vi "FitCurveCorrelation.vi"() -> ()   [LabVIEW 2010]
uses:
  <vilib>/Analysis/1siggen.llb/Ramp Pattern by Samples.vi
  <vilib>/gmath/NumericalOptimization/Nonlinear Curve Fit LM.vi
  <vilib>/gmath/NI_Gmath.lvlib
  <vilib>/Analysis/NI_AALBase.lvlib
panel:
  out "error out":errorcluster
  out "Correlation Matrix":string[][](table)
  out "BestFit":cluster{"Name":string, "Parameter":dbl}[](array[cluster]) caption="Parameter Name          best Fit" {"Parameter" format="%.6f"}
  in  "Guess":T1(array[cluster])=[{"Name"="Offset", "Value"=0.0, "Fit?"=TRUE}, {"Name"="Ampl. 1", "Value"=2.0, "Fit?"=TRUE}, {"Name"="TC 1", "Value"=0.1, "Fit?"=TRUE}, {"Name"="Ampl. 2", "Value"=2.0, "Fit?"=TRUE}, {"Name"="TC 2", "Value"=0.3, "Fit?"=TRUE}] caption="Parameter Name     Guess        Fit?"
  in  "Noise":dbl=0.02
  in  "Simulation parameters":dbl[](array[numeric])=[0.2, 2.0, 0.02, 1.5, 0.2] caption="Offset\n\nAmplitude 1\n\nTime constant 1\n\nAmplitude 2\n\nTime  constant 2"
  in  "stop":bool
  out "XY Graph":cluster{cdb[]}[](graph)
  # "This demo simulates noisy data\nReplace with your experimental data!"
  # "- Run VI\n- Change simulation parameters\n- Change Noise\n- Change Guess\n- enable or disable fitting for some\n   parameters\n\n- Watch the quality of the fit."
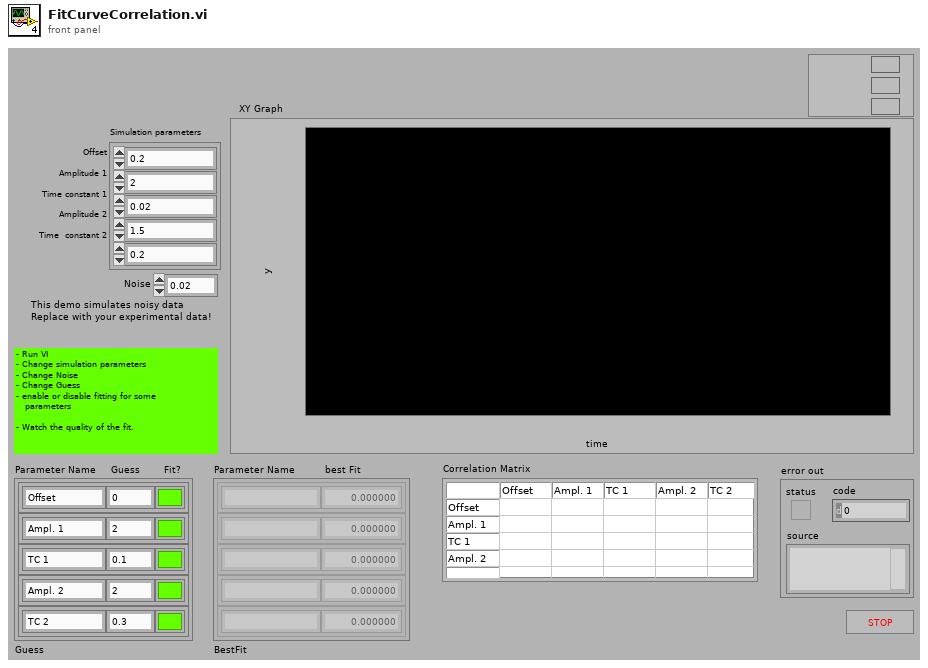
[diagram p1: front panel]
types:
  T1 = cluster{"Name":string, "Value":dbl, "Fit?":bool}[]
  T2 = typedef "NI_Matrix.lvlib/RealMatrix.ctl" = dbl[][]
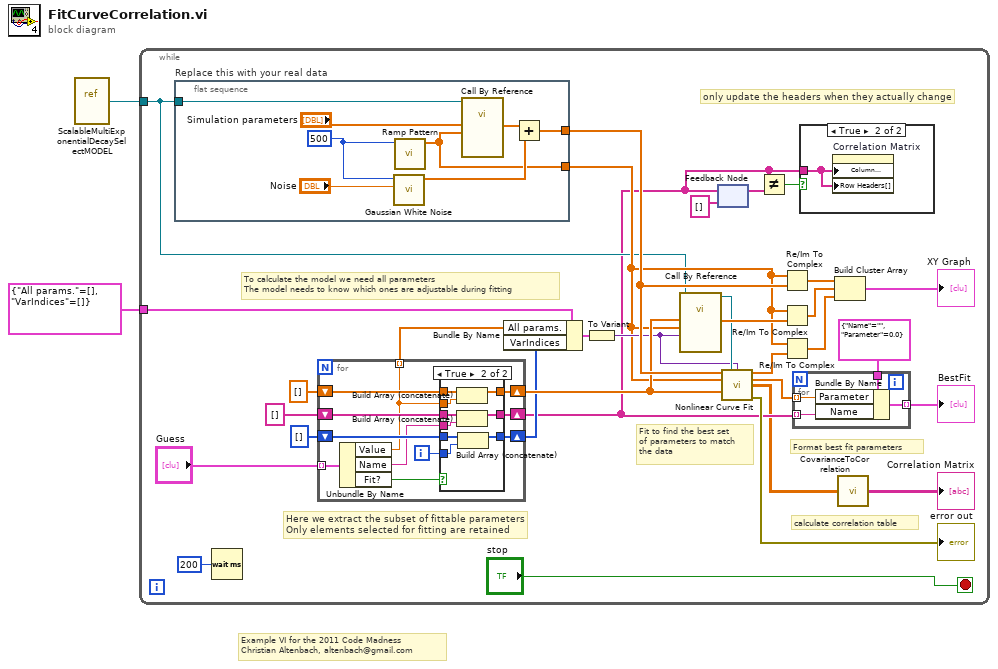
[diagram p0: block diagram]
diagram:
  # "Example VI for the 2011 Code Madness\nChristian Altenbach, altenbach@gmail.com"
  n1 = vi-ref "ScalableMultiExponentialDecaySelectMODEL.vi"() -> (w2:refnum<vi>)
  n2 = while {
    tunnel: w2 -> [w11]
    tunnel: cluster{"All params.":dbl[], "VarIndices":i32[]} {"All params."=[], "VarIndices"=[]} -> [w10]
    stop <- "stop" stop-if-true
    # "calculate correlation table"
    # "only update the headers when they actually change"
    # "Fit to find the best set\nof parameters to match\nthe data"
    # "Format best fit parameters"
    # "To calculate the model we need all parameters\nThe model needs to know which ones are adjustable during fitting"
    # "Here we extract the subset of fittable parameters\nOnly elements selected for fitting are retained"
    n3 = flat-sequence "Replace this with your real data" {
      tunnel: [w39] -> w25
      tunnel: [w37] -> w12
      tunnel: w11 -> [w36]
      frame #0 {
        w43 = 500 ("samples")
        n4 = call <vilib>:"Gaussian White Noise.vi"("standard deviation"="Noise", "samples"=w43) -> ("Gaussian noise pattern"=w41:dbl[])  [unwired: 8 in, 1 out]
        n5 = call-poly <vilib>:"Ramp Pattern.vi"("samples"=w43) -> ("Ramp Pattern"=w37:dbl[])  [unwired: 9 in, 1 out]
        n6 = call-by-ref "?"(reference=w36, "frequency"=w37, "tau"="Simulation parameters") -> ("Phase"=w42:dbl[])  [unwired: 3 in, 4 out]
        n7 = Add(x=w42, y=w41) -> (x+y=w39:dbl[])
      }
    }
    n8 = Wait (ms)(milliseconds to wait=u32 200) -> ()  [unwired: 1 out]
    n9 = for {
      shift-right: [w58] -> w23
      shift-left: dbl[] [] -> [w57]
      tunnel: "Guess" -> [w56] mode=indexing
      tunnel: [w49] -> w20 mode=indexing
      shift-right: [w54] -> w19
      shift-left: i32[] [] -> [w53]
      shift-right: [w50] -> w5
      shift-left: string[] [] -> [w51]
      i -> [w52]
      n10 = Unbundle By Name(w56) -> ("Value"=w49:dbl, "Name"=w48:string, "Fit?"=w55:bool)
      n11 = case shown="True" w55 {
        tunnel: [w61 w69] -> w58
        tunnel: w57 -> [w61 w70]
        tunnel: w49 -> [_ w68]
        tunnel: [w60 w67] -> w54
        tunnel: w53 -> [w60 w66]
        tunnel: w52 -> [_ w65]
        tunnel: [w59 w63] -> w50
        tunnel: w51 -> [w59 w64]
        tunnel: w48 -> [_ w62]
        frame False {
        }
        frame True {
          n12 = Build Array (concatenate)(w70, w68) -> (w69:dbl[])
          n13 = Build Array (concatenate)(w64, w62) -> (w63:string[])
          n14 = Build Array (concatenate)(w66, w65) -> (w67:i32[])
        }
      }
    }
    n15 = Bundle By Name(cluster=w10, "All params."=w20, "VarIndices"=w19) -> (w24:cluster{"All params.":dbl[], "VarIndices":i32[]})
    n16 = To Variant(anything=w24) -> (Variant=w17:variant)
    n17 = call-by-ref "?"(reference=w11, "data"=w17, "frequency"=w12, "tau"=w23) -> (reference out=w28:refnum<vi>, "Phase"=w29:dbl[])  [unwired: 2 in, 3 out]
    n18 = feedback-in #1(w5) -> ()
    n19 = feedback #1(string[] []) -> (w8:string[])
    n20 = call-poly <vilib>:"Nonlinear Curve Fit.vi"("Y"=w25, "f(x,a)"=w28, "data"=w17, "X"=w12, "initial parameters"=w23) -> ("best nonlinear fit"=w32:dbl[], "best fit parameters"=w15:dbl[], "covariance"=w4:T2, "error out"=→"error out":errorcluster)  [unwired: 5 in, 2 out]
    n21 = Not Equal?(x=w5, y=w8) -> (x != y?=w6:bool)
    n22 = Re/Im To Complex(1:w25, 2:w12) -> (0:w34:cdb[])
    n23 = Re/Im To Complex(1:w29, 2:w12) -> (0:w31:cdb[])
    n24 = Re/Im To Complex(1:w32, 2:w12) -> (0:w30:cdb[])
    n25 = for {
      tunnel: w5 -> [w45] mode=indexing
      tunnel: w15 -> [w47] mode=indexing
      tunnel: cluster{"Name":string, "Parameter":dbl} {"Name"="", "Parameter"=0.0} -> [w46]
      tunnel: [w44] -> w13 mode=indexing
      n26 = Bundle By Name(cluster=w46, "Parameter"=w47, "Name"=w45) -> (w44:cluster{"Name":string, "Parameter":dbl})
    }
    "BestFit" <- w13
    n27 = case shown="True" w6 {
      tunnel: w5 -> [_ w35]
      frame False {
      }
      frame True {
        n28 = property on="Correlation Matrix" class="Tbl (strict)"("Column Headers[]"=w35, "Row Headers[]"=w35) -> ()  [unwired: 2 in, 2 out]
      }
    }
    n29 = Build Cluster Array(w34, w31, w30) -> (→"XY Graph":cluster{cdb[]}[])
    n30 = call "CovarianceToCorrelation.vi"("covariance matrix"=w4) -> ("Correlation table"=→"Correlation Matrix":string[][])
  }
